vi "Main.vi"() -> ()   [LabVIEW 2020]
uses:
  <vilib>/DAQmx/read.llb/DAQmx Read (Analog DBL 1Chan 1Samp).vi
  <vilib>/DAQmx/create/channels.llb/DAQmx Create Channel (AI-Temperature-Thermocouple).vi
  <vilib>/DAQmx/configure/timing.llb/DAQmx Timing (Sample Clock).vi
  <vilib>/DAQmx/miscellaneous.llb/DAQmx Fill In Error Info.vi
panel:
  in  "maximum value":dbl=100.0 format="%#_13g"
  in  "minimum value":dbl format="%#_13g"
  in  "Stop":bool
  out "Waveform Chart":dbl(graph)
  in  "Thermocouple Channel":tag="PCI-6221/ai0"
  # "Measurement Range (deg C)"
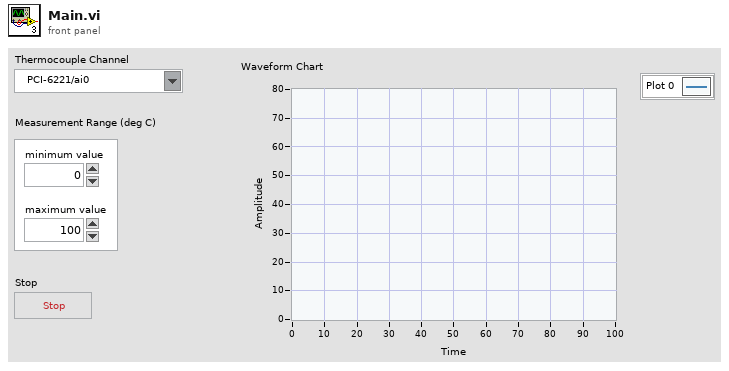
[diagram p1: front panel]
types:
  T1 = enum16{"open", "replace", "create", "open or create", "replace or create", "replace or create with confirmation"}
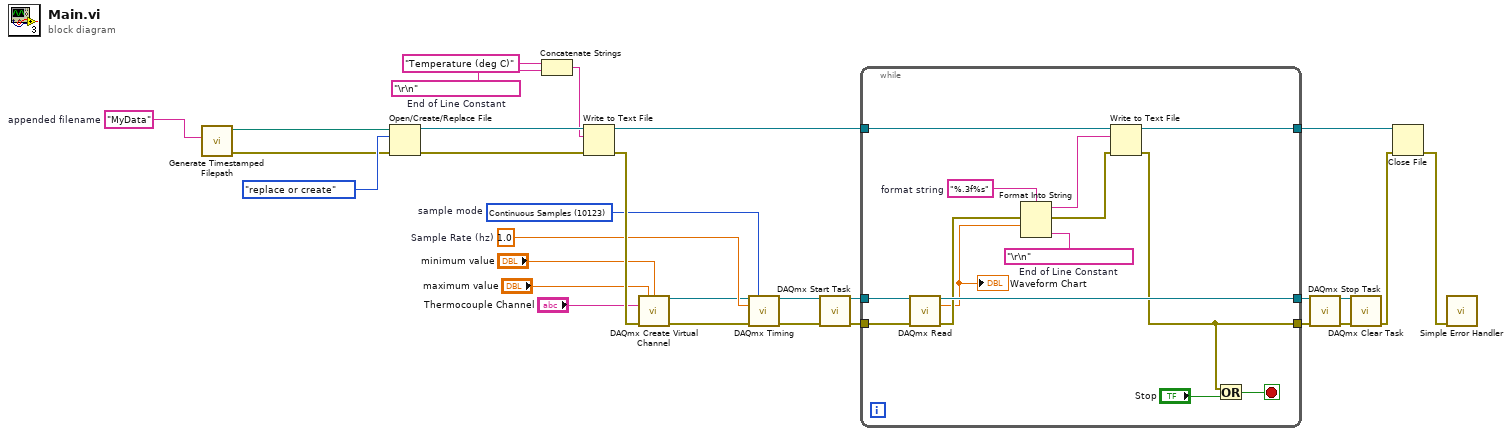
[diagram p0: block diagram]
diagram:
  w1 = "MyData"  # appended filename
  w13 = "\r\n"  # End of Line Constant
  w27 = 1.0  # Sample Rate (hz)
  w28 = 10123 items=["Finite Samples"=10178, "Continuous Samples"=10123, "Hardware Timed Single Point"=12522]  # sample mode
  n1 = call "Generate Timestamped Filepath.vi"("appended filename"=w1) -> ("Error Out"=w2:errorcluster, "timestamped relative filepath"=w3:path)  [unwired: 9 in]
  n2 = Open/Create/Replace File(file path (use dialog)=w3, error in=w2, operation (0:open)=T1."replace or create") -> (refnum out=w16:refnum<file>, error out=w15:errorcluster)  [unwired: 3 in, 1 out]
  n3 = Concatenate Strings("Temperature (deg C)" ("string"), w13) -> (w12:string)
  n4 = Write to Text File(file (use dialog)=w16, text=w12, error in=w15) -> (refnum out=w11:refnum<file>, error out=w29:errorcluster)  [unwired: 1 in, 1 out]
  n5 = call-poly <vilib>:"DAQmx Create Virtual Channel.vi"("maximum value"="maximum value", "minimum value"="minimum value", "physical channels"="Thermocouple Channel", "error in"=w29) -> ("task out"=w26:refnum<k21>, "error out"=w25:errorcluster)  [unwired: 10 in]
  n6 = call-poly <vilib>:"DAQmx Timing.vi"("task/channels in"=w26, "sample mode"=w28, "rate"=w27, "error in"=w25) -> ("task out"=w24:refnum<k21>, "error out"=w23:errorcluster)  [unwired: 10 in]
  n7 = call <vilib>:"DAQmx Start Task.vi"("task/channels in"=w24, "error in"=w23) -> ("task out"=w19:refnum<k21>, "error out"=w18:errorcluster)  [unwired: 12 in]
  n8 = while {
    tunnel: [w43] -> w10
    tunnel: w19 -> [w40]
    tunnel: w18 -> [w39]
    tunnel: w11 -> [w32]
    tunnel: [w31] -> w9
    tunnel: [w30] -> w5
    stop <- w41 stop-if-true
    w35 = "%.3f%s"  # format string
    w38 = "\r\n"  # End of Line Constant
    n9 = call-poly <vilib>:"DAQmx Read.vi"("task/channels in"=w40, "error in"=w39) -> ("task out"=w43:refnum<k21>, "data"=w36:dbl, "error out"=w37:errorcluster)  [unwired: 11 in]
    "Waveform Chart" <- w36
    n10 = Format Into String(format string=w35, error in=w37, w36, w38) -> (resulting string=w34:string, error out=w33:errorcluster)  [unwired: 1 in]
    n11 = Write to Text File(file (use dialog)=w32, text=w34, error in=w33) -> (refnum out=w30:refnum<file>, error out=w31:errorcluster)  [unwired: 1 in, 1 out]
    n12 = Or(x=w31, y="Stop") -> (x .or. y?=w41:bool)
  }
  n13 = call <vilib>:"DAQmx Stop Task.vi"("task/channels in"=w10, "error in"=w9) -> ("task out"=w8:refnum<k21>, "error out"=w7:errorcluster)  [unwired: 12 in]
  n14 = call <vilib>:"DAQmx Clear Task.vi"("task in"=w8, "error in"=w7) -> ("error out"=w6:errorcluster)  [unwired: 13 in]
  n15 = Close File(refnum=w5, error in=w6) -> (error out=w4:errorcluster)  [unwired: 1 out]
  n16 = call <vilib>:"Simple Error Handler.vi"("error in (no error)"=w4) -> ()  [unwired: 4 in, 5 out]
